vi "test_gen.vi"() -> ()   [LabVIEW 2018]
panel:
  out "数组":dbl[](array[numeric])
  in  "观测时刻（0-1）":dbl[](array[numeric])
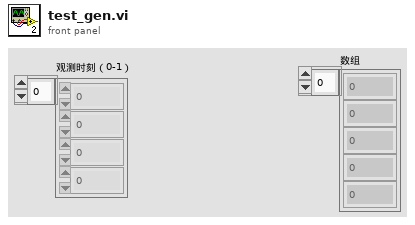
[diagram p1: front panel]
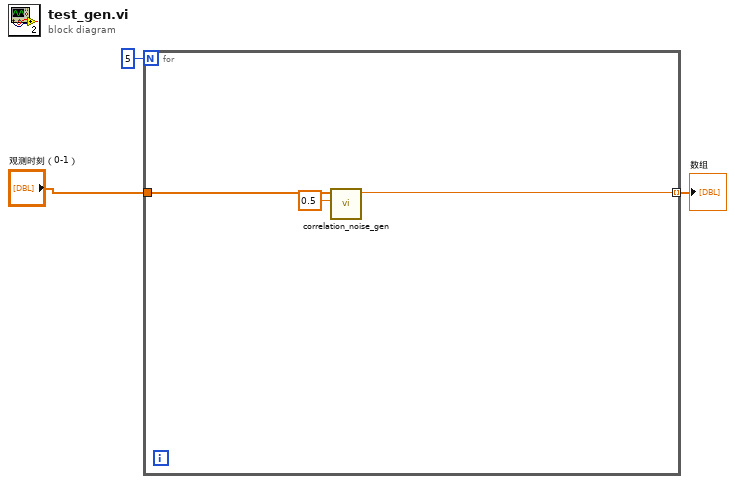
[diagram p0: block diagram]
diagram:
  n1 = for {
    N: 5 -> [_]
    tunnel: "观测时刻（0-1）" -> [w6]
    tunnel: [w4] -> w1 mode=indexing
    n2 = call "correlation_noise_gen.vi"("噪声方差"=0.5, "观测时刻（0-1）"=w6) -> ("平均观测噪声"=w4:dbl)  [unwired: 9 in]
  }
  "数组" <- w1
